vi "Write Encoding.vi"(8 "error in (no error)":errorcluster, 10 "Encoding":T1, 11 "SQL Statement in":refnum<class "SQL Statement.lvclass">) -> (0 "error out":errorcluster, 3 "SQL Statement out":refnum<class "SQL Statement.lvclass">)   [LabVIEW 2023, in "SQLiteSupport.lvlib" / "SQL Statement.lvclass"]
doc: "Text encoding for Bind Text and Get Column Text.\n1) System -- Assumed to be the system encoding used by LabVIEW. Text is converted to UTF-8 before being passed to SQLite, and UTF-8 results from SQLite are coverted back the the system encoding.\n2) UTF-8 -- Strings assumed to be UTF-8. Note that ASCII is a valid subset of UTF-8.\n3) UTF-16 -- Strings assumed to be UTF-16.\n\nNote that encoding does not affect BLOB binary data."
uses:
  SQL Statement.lvclass
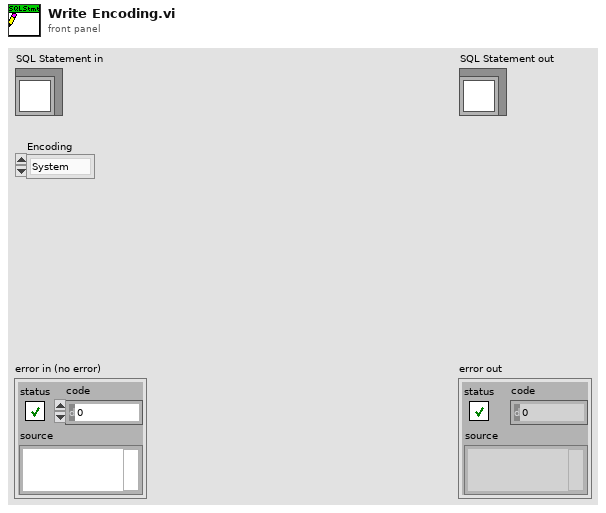
[diagram p1: front panel]
types:
  T1 = typedef "SQLiteSupport.lvlib/SQL Statement.lvclass/Text Encoding" = enum16{"System", "UTF-8", "UTF-16"}
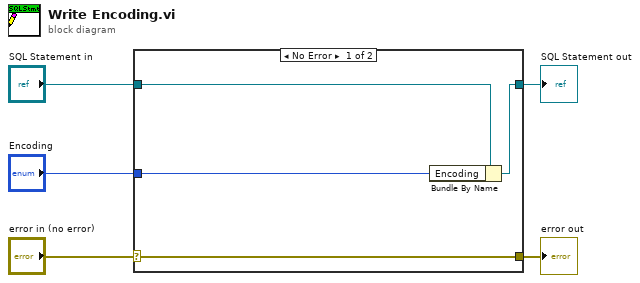
[diagram p0: block diagram]
diagram:
  n1 = case shown="No Error" "error in (no error)" {
    selector: "error in (no error)" -> [w9 w10]
    tunnel: [w9 w10] -> w4
    tunnel: [w7 w11] -> w2
    tunnel: "SQL Statement in" -> [w8 w11]
    tunnel: "Encoding" -> [w6 _]
    frame No Error {
      n2 = Bundle By Name(cluster=w8, "Encoding"=w6) -> (w7:refnum<class "SQL Statement.lvclass">)
    }
    frame Error {
    }
  }
  "error out" <- w4
  "SQL Statement out" <- w2
